vi "MainTranslator.vi"() -> ()   [LabVIEW 2024]
panel:
  out "Array":path[](array[path])
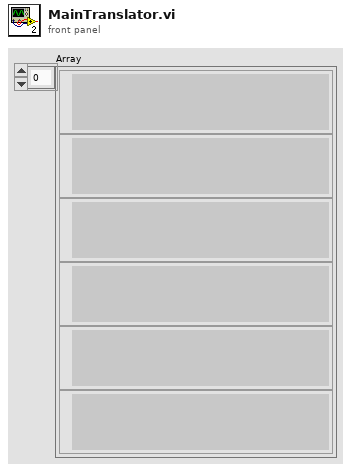
[diagram p1: front panel]
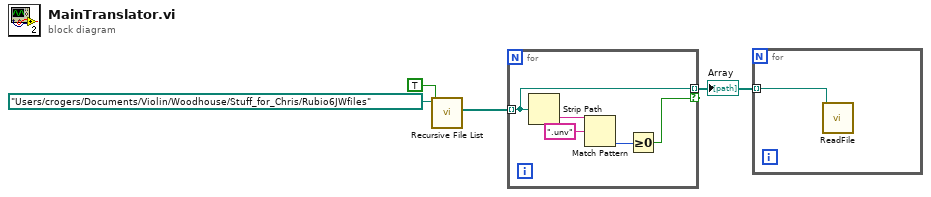
[diagram p0: block diagram]
diagram:
  n1 = call <vilib>:"Recursive File List.vi"("Continue Recursing on Error? (F)"=TRUE, "Folder Path"=path "/Users/crogers/Documents/Violin/Woodhouse/Stuff_for_Chris/Rubio6JWfiles") -> ("All Files in Dir"=w2:path[])  [unwired: 5 in, 4 out]
  n2 = for {
    tunnel: w2 -> [w7] mode=indexing
    tunnel: [w7] -> w1 mode=indexing if=w5
    n3 = Strip Path(path=w7) -> (name=w9:string)  [unwired: 1 out]
    n4 = Match Pattern(string=w9, regular expression=".unv") -> (offset past match=w6:i32)  [unwired: 1 in, 3 out]
    n5 = Greater Or Equal To 0?(x=w6) -> (x >= 0?=w5:bool)
  }
  "Array" <- w1
  n6 = for {
    tunnel: w1 -> [w10] mode=indexing
    n7 = call "ReadFile.vi"("UFF Path"=w10) -> ()  [unwired: 10 in, 1 out]
  }
